vi "test Receive Message Abort.vi"(8 "error in (no error)":errorcluster, 11 "TestCase in":refnum<class "Test TCP Stream Transmission.lvclass">) -> (0 "error out":errorcluster, 3 "TestCase out":refnum<class "Test TCP Stream Transmission.lvclass">)   [LabVIEW 2020, in "Test TCP Stream Transmission.lvclass"]
uses:
  Test TCP Stream Transmission.lvclass
  <vilib>/addons/_JKI Toolkits/VI Tester/TestCase.llb/TestCase.lvclass
  Source/Protocols/TCP Strategy/TCP Stream Initiator/TCP Stream Initiator.lvclass
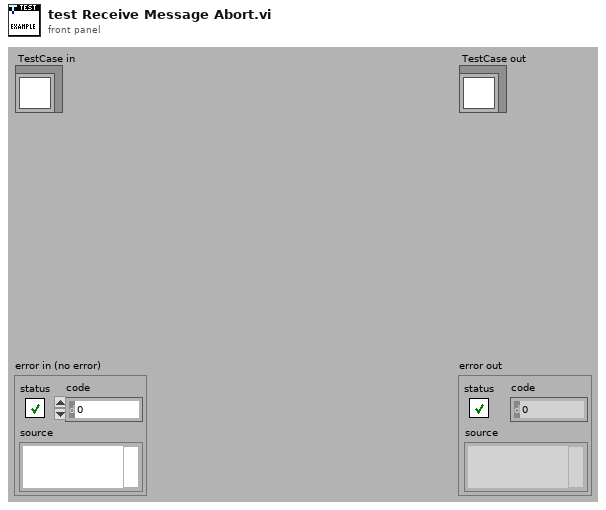
[diagram p1: front panel]
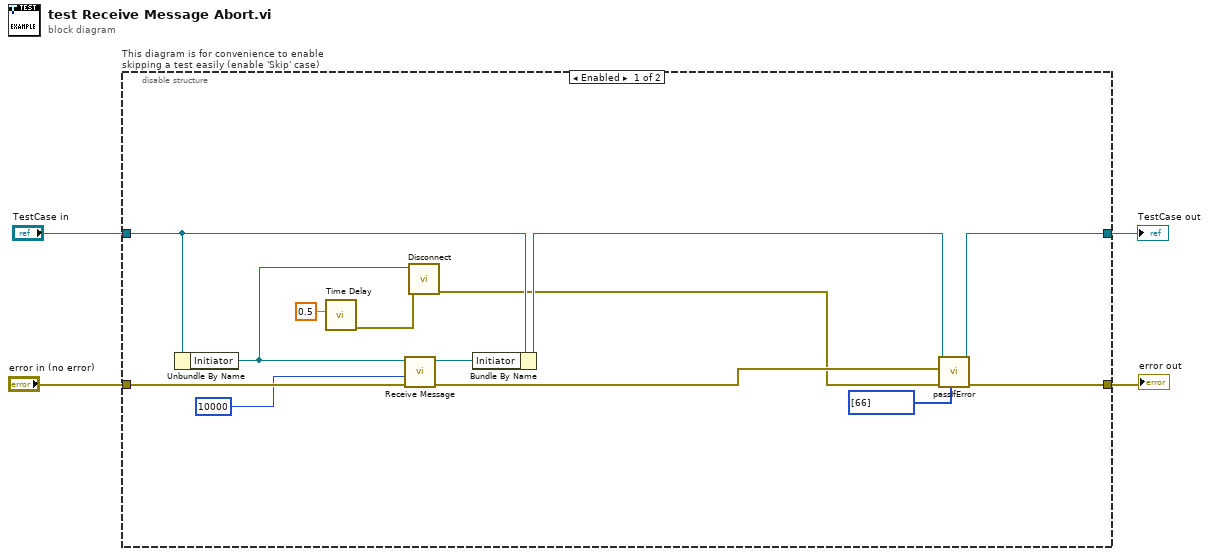
[diagram p0: block diagram]
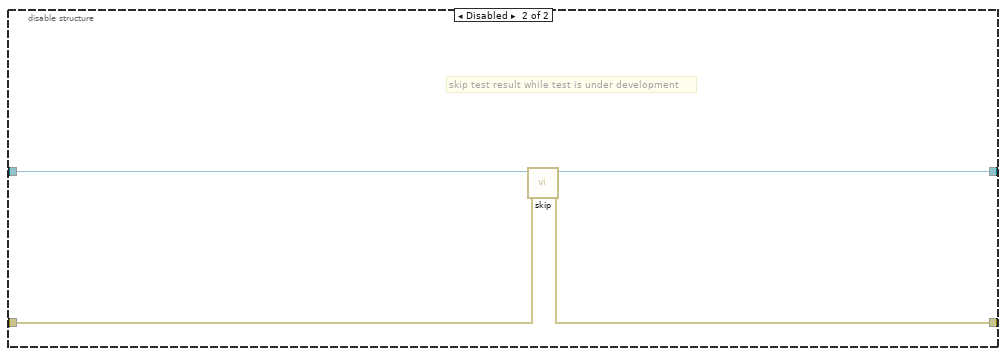
[diagram p2: hidden frame]
diagram:
  n1 = disable-structure "This diagram is for convenience to enable skipping a test easily (enable 'Skip' case)" shown="Enabled" {
    disable-tunnel: "TestCase in" -> [w13 w21]
    disable-tunnel: [w17 w19] -> w3
    disable-tunnel: [w16 w20] -> w1
    disable-tunnel: "error in (no error)" -> [w15 w18]
    frame Enabled {
      n2 = Unbundle By Name(w13) -> ("Initiator"=w8:refnum<class "TCP Stream Initiator.lvclass">)
      n3 = call "Time Delay"("Delay Time (s)"=0.5) -> ("error out"=w6:errorcluster)  [unwired: 10 in]
      n4 = call-dynamic "Receive Message.vi"("error in (no error)"=w15, "timeout ms (-1)"=10000, "TCP Stream in"=w8) -> ("error out"=w10:errorcluster, "TCP Stream out"=w14:refnum<class "TCP Stream Initiator.lvclass">)  [unwired: 4 in, 3 out]
      n5 = call-dynamic "Disconnect.vi"("error in (no error)"=w6, "TCP Stream in"=w8) -> ("error out"=w5:errorcluster)  [unwired: 8 in, 1 out]
      n6 = Bundle By Name(cluster=w13, "Initiator"=w14) -> (w12:refnum<class "Test TCP Stream Transmission.lvclass">)
      n7 = call-dynamic "passIfError.vi"("passing error codes (default = any error code)"=i32[] [66], "error in (no error)"=w5, "error"=w10, "TestCase in"=w12) -> ("error out"=w16:errorcluster, "TestCase out"=w17:refnum<class "Test TCP Stream Transmission.lvclass">)  [unwired: 6 in]
    }
    frame Disabled {
      # "skip test result while test is under development"
      n8 = call <vilib>:"skip.vi"("error in (no error)"=w18, "TestCase in"=w21) -> ("error out"=w20:errorcluster, "TestCase out"=w19:refnum<class "Test TCP Stream Transmission.lvclass">)  [unwired: 8 in]
    }
  }
  "error out" <- w1
  "TestCase out" <- w3
